vi "Pockels-Force modulation ON.vi"(8 "error in (no error)":errorcluster) -> (0 "error out":errorcluster)   [LabVIEW 2020]
uses:
  Global Variables/General Globals.vi
  Globals/gl_Pockels control globals.vi
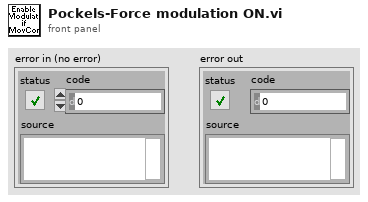
[diagram p1: front panel]
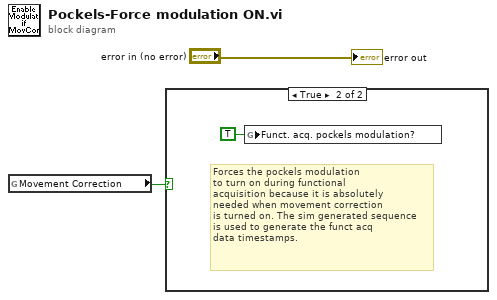
[diagram p0: block diagram]
diagram:
  n1 = global read "General Globals.vi" "Movement Correction"() -> (w1:bool)
  n2 = case shown="True" w1 {
    frame False {
    }
    frame True {
      # "Forces the pockels modulation\nto turn on during functional\nacquisition because it is absolutely\nneeded when movement correction\nis turned on. The sim generated sequence\nis used to generate the funct acq \ndata timestamps."
      n3 = global write "gl_Pockels control globals.vi" "Funct. acq. pockels modulation?"(TRUE ("Pockels modulation is ON")) -> ()
    }
  }
  "error out" <- "error in (no error)"
